vi "SLSC Get All Channels.vi"(6 "SLSCChannelPath":string="SLSCChannelPath", 8 "error in (no error)":errorcluster, 11 "Item Ref in":T1 format="%.0x") -> (0 "error out":errorcluster, 1 "Channel Values":dbl[](array[numeric]), 2 "TreeItem Channels":string[](array[string]), 3 "Item Ref out":T1 format="%.0x")   [LabVIEW 2020, in "SLSC CD System Explorer.lvlib"]
uses:
  SLSC CD System Explorer.lvlib
  <vilib>/NI VeriStand/Custom Device API/Custom Device Item Ref.ctl
  <vilib>/NI VeriStand/Custom Device API/Get Item Property (String).vi
  <vilib>/NI VeriStand/Custom Device Tools/Custom Device Utility Library/Custom Device Utility Library.lvlib
  <vilib>/NI VeriStand/Custom Device API/Custom Device API.lvlib
  SLSC CD Shared/SLSC CD Shared.lvlib
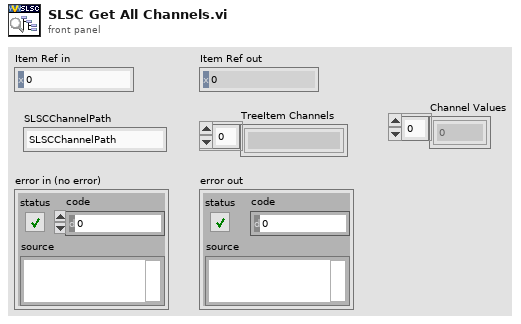
[diagram p1: front panel]
types:
  T1 = typedef "Custom Device API.lvlib/Custom Device Item Ref.ctl" = u64
  T2 = typedef "Custom Device API.lvlib/Custom Device Channel.ctl" = cluster{"Type":T3, "Units":string, "Default Value":dbl, "Faultable":bool, "Scalable":bool}
  T3 = typedef "Custom Device API.lvlib/Custom Device Channel Type.ctl" = enum16{"Input", "Output"}
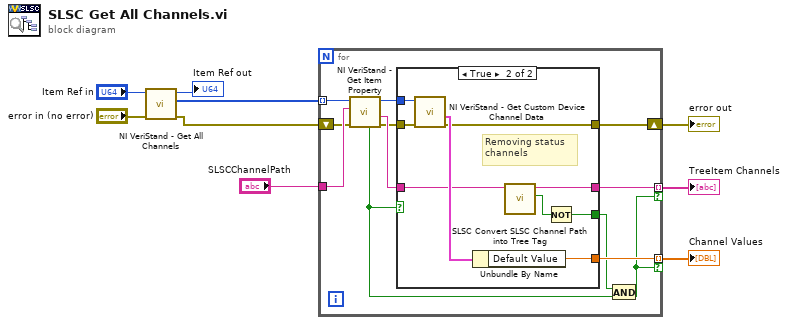
[diagram p0: block diagram]
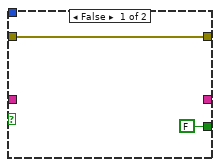
[diagram p2: hidden frame]
diagram:
  n1 = call <vilib>:"NI VeriStand - Get All Channels.vi"("error in"="error in (no error)", "Section Ref in"="Item Ref in") -> ("error out"=w4:errorcluster, "Channel Refs"=w6:T1[], "Section Ref out"=→"Item Ref out":T1)  [unwired: 6 in, 1 out]
  n2 = for {
    tunnel: w6 -> [w17] mode=indexing
    tunnel: "SLSCChannelPath" -> [w21]
    tunnel: [w19] -> w7 mode=indexing if=w11
    tunnel: [w12] -> w3 mode=indexing if=w11
    shift-right: [w13] -> w2
    shift-left: w4 -> [w18]
    n3 = call-poly <vilib>:"NI VeriStand - Get Item Property.vi"("error in (no error)"=w18, "Property Name"=w21, "Item Ref in"=w17) -> ("error out"=w14:errorcluster, "Value"=w20:string, "Item Ref out"=w15:T1, "Found?"=w16:bool)  [unwired: 5 in]
    n4 = case shown="True" w16 {
      tunnel: w20 -> [_ w26]
      tunnel: [_ w32] -> w19
      tunnel: w15 -> [_ w30]
      tunnel: w14 -> [w23 w29]
      tunnel: [w23 w27] -> w13
      tunnel: [_ w28] -> w12
      tunnel: [FALSE w24] -> w10
      frame False {
      }
      frame True {
        # "Removing status \nchannels"
        n5 = call <vilib>:"NI VeriStand - Get Custom Device Channel Data.vi"("error in (no error)"=w29, "Channel Ref in"=w30) -> ("error out"=w27:errorcluster, "Channel"=w31:T2)  [unwired: 4 in, 4 out]
        n6 = Unbundle By Name(w31) -> ("Default Value"=w28:dbl)
        n7 = call "SLSC Convert SLSC Channel Path into Tree Tag.vi"("SLSC Channel Path"=w26) -> ("Status?"=w25:bool, "Tree Item Channel"=w32:string)  [unwired: 9 in]
        n8 = Not(x=w25) -> (.not. x?=w24:bool)
      }
    }
    n9 = And(x=w10, y=w16) -> (x .and. y?=w11:bool)
  }
  "error out" <- w2
  "TreeItem Channels" <- w7
  "Channel Values" <- w3
